vi "Write Source Channels.vi"(8 "error in (no error)":errorcluster, 10 "Source Channels":string[](array[string]), 11 "%DEVICE% Init Parameters in":refnum<class "%DEVICE% Init Parameters.lvclass">) -> (0 "error out":errorcluster, 3 "%DEVICE% Init Parameters out":refnum<class "%DEVICE% Init Parameters.lvclass">)   [LabVIEW 2017, in "%DEVICE% Messaging.lvlib" / "%DEVICE% Init Parameters.lvclass"]
uses:
  %DEVICE% Init Parameters.lvclass
  %DEVICE% Init Parameters.lvclass/%DEVICE% Init Parameters.ctl
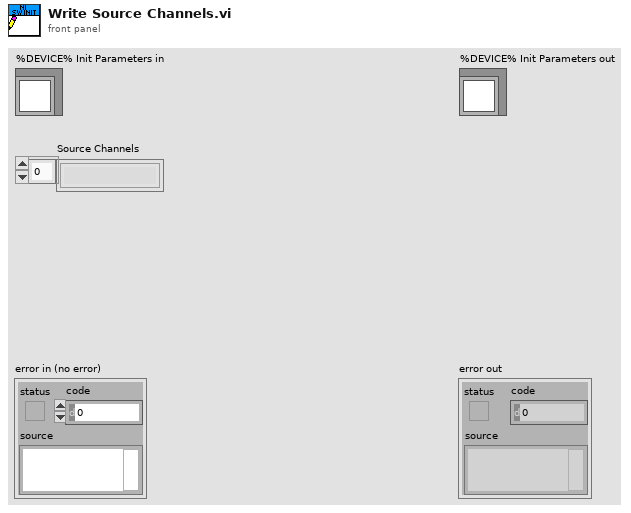
[diagram p1: front panel]
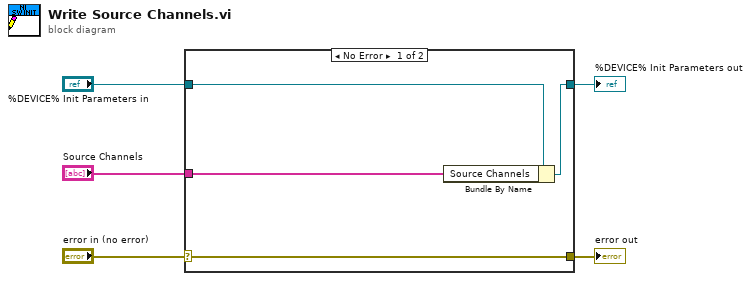
[diagram p0: block diagram]
diagram:
  n1 = case shown="No Error" "error in (no error)" {
    selector: "error in (no error)" -> [w9 w10]
    tunnel: [w9 w10] -> w4
    tunnel: [w7 w11] -> w2
    tunnel: "%DEVICE% Init Parameters in" -> [w8 w11]
    tunnel: "Source Channels" -> [w6 _]
    frame No Error {
      n2 = Bundle By Name(cluster=w8, "Source Channels"=w6) -> (w7:refnum<class "%DEVICE% Init Parameters.lvclass">)
    }
    frame Error {
    }
  }
  "error out" <- w4
  "%DEVICE% Init Parameters out" <- w2
